vi "New.vi"(8 "error in (no error)":errorcluster) -> (0 "error out":errorcluster, 3 "TipPanelHandle out":refnum<class "TipPanelHandle.lvclass">)   [LabVIEW 2021, in "TipStripOOPanel.lvlib" / "TipPanelHandle.lvclass"]
uses:
  TipPanelHandle.lvclass
  TipPanelHandle.lvclass/TipPanelHandle.ctl
  TipPanel/TipPanel.lvclass
  SubVIs/tipstrip action.ctl
  TipStripOOPanel.lvlib
  SubVIs/tipstrip UE data.ctl
  TipStrip Daemon.vi
  <vilib>/Futures/Futures/Promise/Promise.lvclass
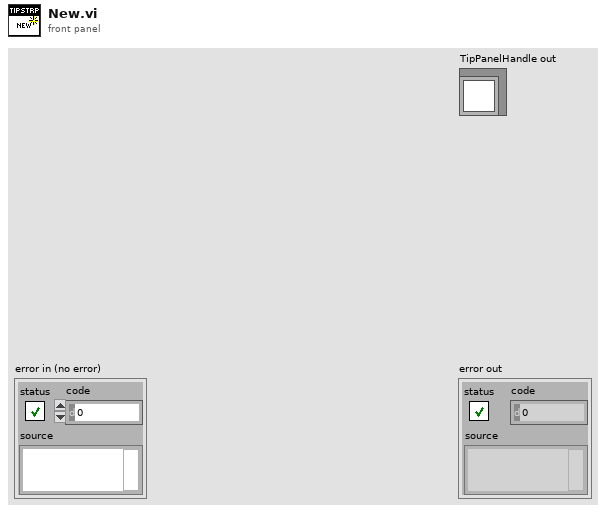
[diagram p1: front panel]
types:
  T1 = typedef "TipStripOOPanel.lvlib/tipstrip UE data.ctl" = cluster{"action":T2, "TipPanel":refnum<class "TipPanel.lvclass">}
  T2 = typedef "TipStripOOPanel.lvlib/tipstrip action.ctl" = enum16{"hide", "show"}
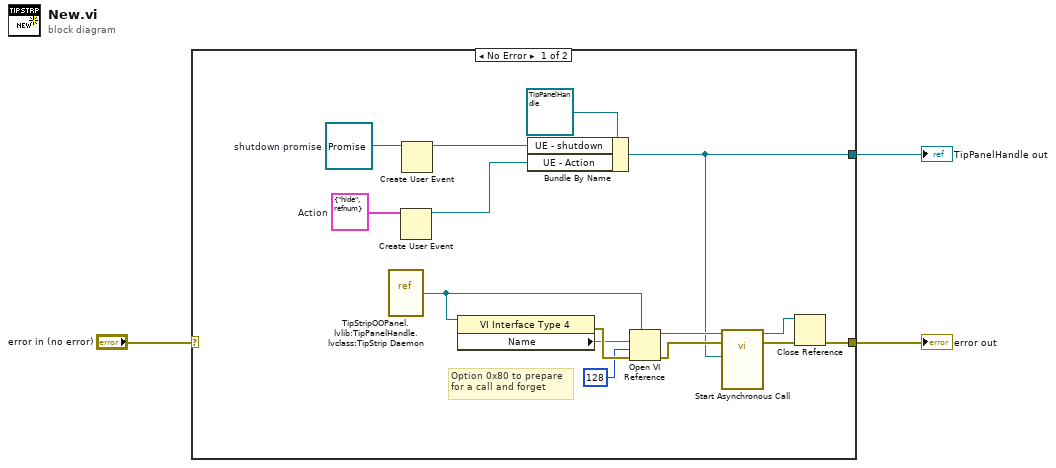
[diagram p0: block diagram]
diagram:
  n1 = case shown="No Error" "error in (no error)" {
    selector: "error in (no error)" -> [_ w19]
    tunnel: [w7 w19] -> w1
    tunnel: [w9 _] -> w3
    frame No Error {
      w5 = refnum<class "Promise.lvclass"> refnum  # shutdown promise
      w10 = T1 {"action"=enum."hide", "TipPanel"=refnum}  # Action
      # "Option 0x80 to prepare\nfor a call and forget"
      n2 = vi-ref "TipStripOOPanel.lvlib:TipPanelHandle.lvclass:TipStrip Daemon.vi"() -> (w17:refnum<vi>)
      n3 = Create User Event(user event datatype=w10) -> (user event=w12:refnum<user-event>)  [unwired: 1 in, 1 out]
      n4 = Create User Event(user event datatype=w5) -> (user event=w4:refnum<user-event>)  [unwired: 1 in, 1 out]
      n5 = property class="VI Interface Type 4"(reference=w17) -> (error out=w15:errorcluster, "Name"=w14:string)  [unwired: 1 in, 1 out]
      n6 = Bundle By Name(cluster=refnum<class "TipPanelHandle.lvclass"> refnum ("TipStripOOPanel.lvlib:TipPanelHandle.lvclass"), "UE - shutdown"=w4, "UE - Action"=w12) -> (w9:refnum<class "TipPanelHandle.lvclass">)
      n7 = Open VI Reference(type specifier VI Refnum (for type only)=w17, vi path=w14, options=128, error in (no error)=w15) -> (vi reference=w16:refnum<vi>, error out=w18:errorcluster)  [unwired: 2 in]
      n8 = call-by-ref "Start Asynchronous Call"(reference=w16, error in=w18, "TipStripOOPanel.lvlib:TipPanelHandle.lvclass"=w9) -> (reference out=w6:refnum<vi>, error out=w8:errorcluster)  [unwired: 11 in]
      n9 = Close Reference(reference=w6, error in (no error)=w8) -> (error out=w7:errorcluster)
    }
    frame Error {
    }
  }
  "error out" <- w1
  "TipPanelHandle out" <- w3
